vi "testclient.vi"() -> ()   [LabVIEW 2016]
uses:
  dllwrapper/tls data user event.ctl
  dllwrapper/tls new socket user event.ctl
  dllwrapper/async tls.lvlib
  lvasynctls.dll
panel:
  out "data 2":string
  out "data":string
  out "connection":u32
  out "errstring":string
  out "request type 3":u8 format="%.0x"
  out "request ID 3":u32 format="%.0x"
  out "error code 3":i32 format="%.0x"
  out "request type 2":u8 format="%.0x"
  out "request ID 2":u32 format="%.0x"
  out "error code 2":i32 format="%.0x"
  out "error code":i32
  out "request ID":u32 format="%.0x"
  out "request type":u32 format="%.0x"
  out "error out 10":errorcluster
  out "error out 9":errorcluster
  out "error out 6":errorcluster
  out "error out 5":errorcluster
  out "error out 4":errorcluster
  out "error out 3":errorcluster
  out "error out 2":errorcluster
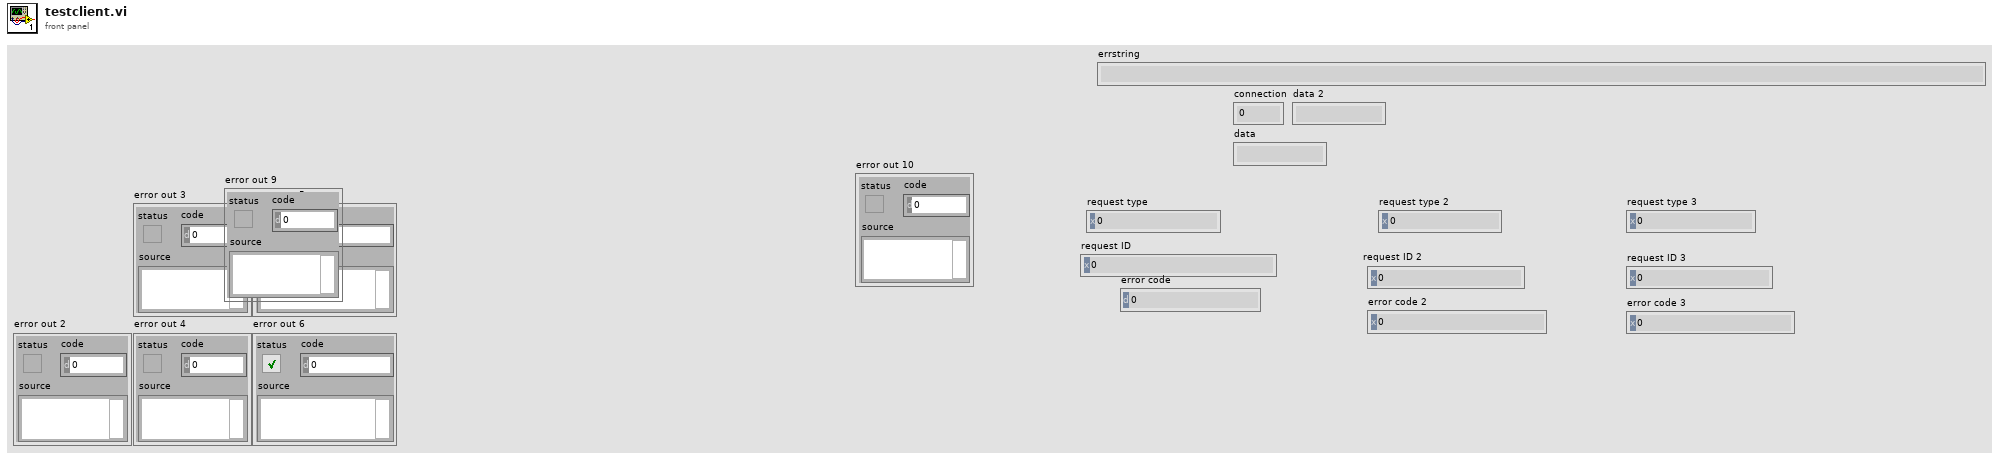
[diagram p1: front panel]
types:
  T1 = typedef "async tls.lvlib/tls new socket user event.ctl" = cluster{"request type":u32, "request ID":u32, "error code":i32, "errstring":string, "connection":u64}
  T2 = typedef "async tls.lvlib/tls data user event.ctl" = cluster{"request type":u8, "request ID":u32, "error code":i32, "data":string}
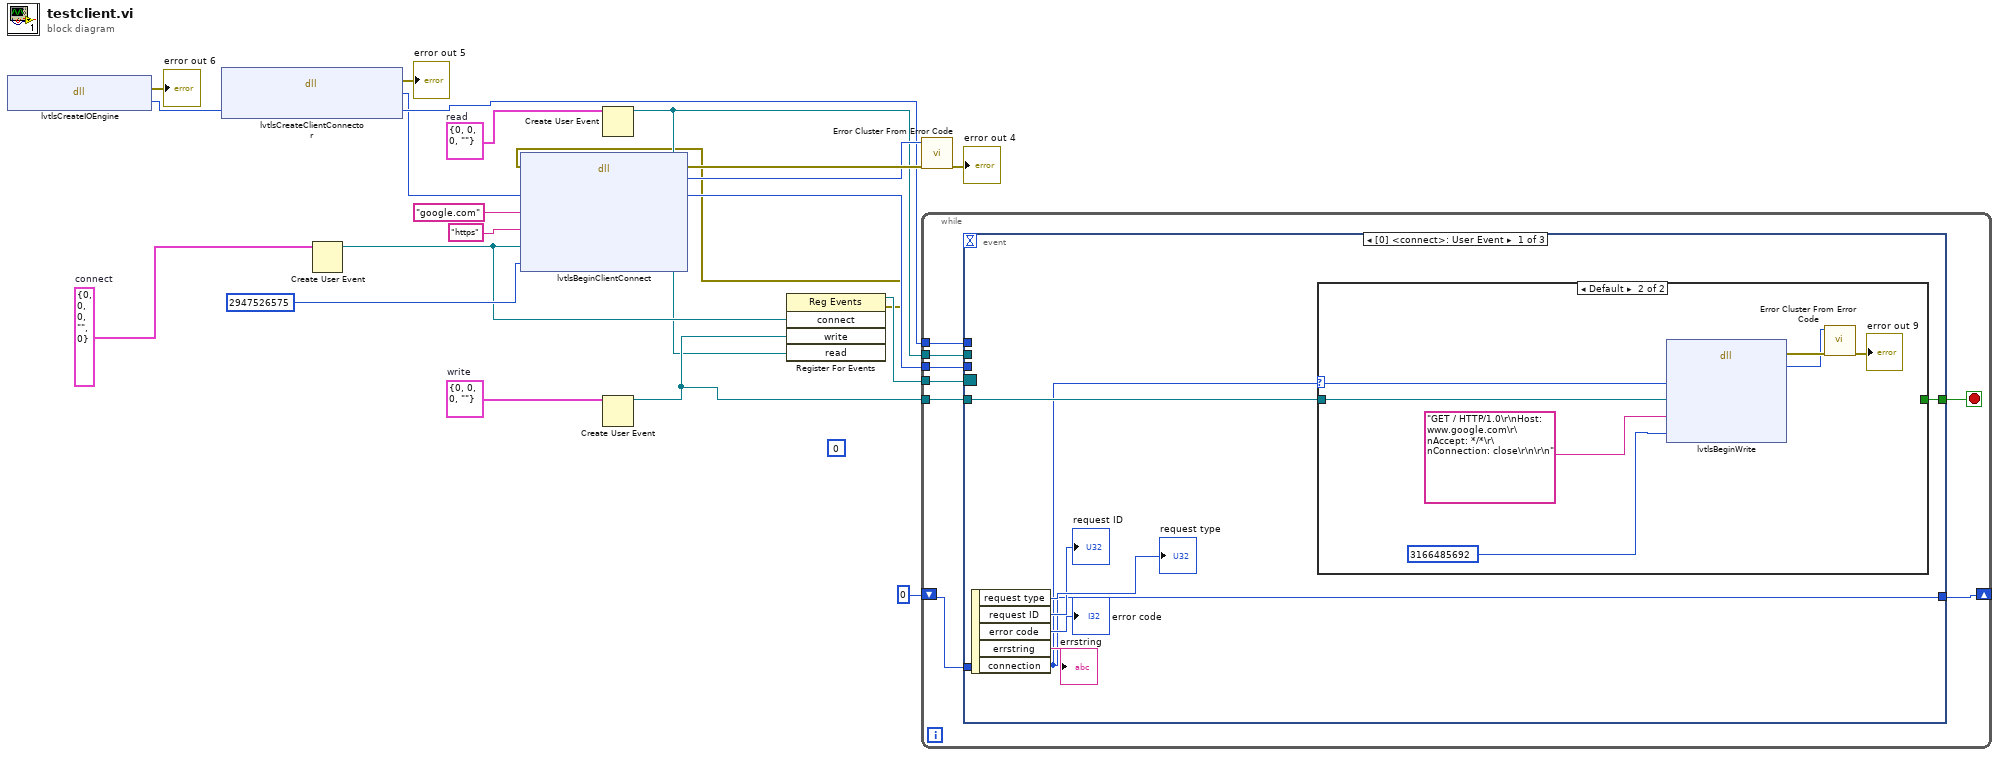
[diagram p0: block diagram]
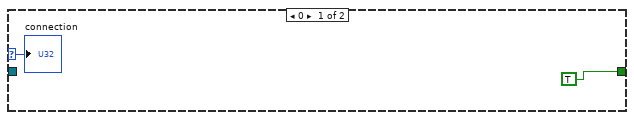
[diagram p2: hidden frame]
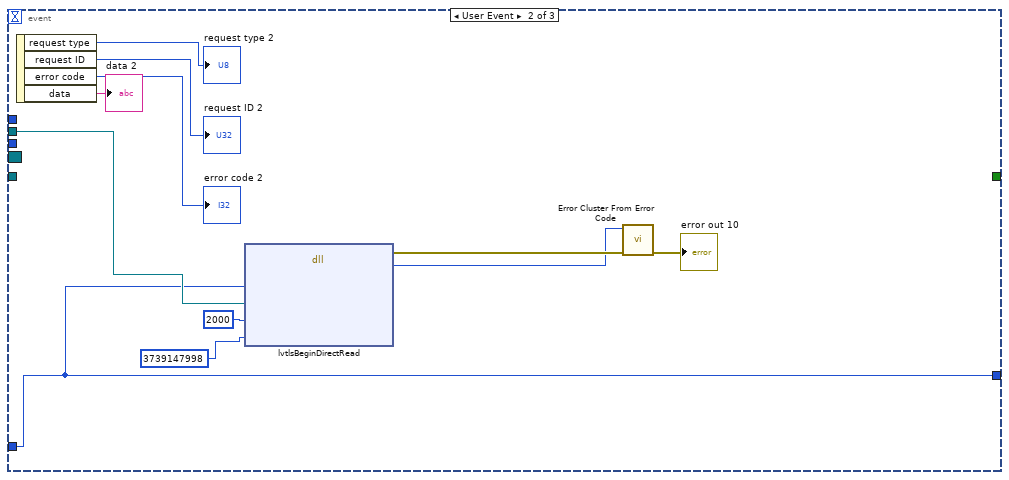
[diagram p3: hidden frame]
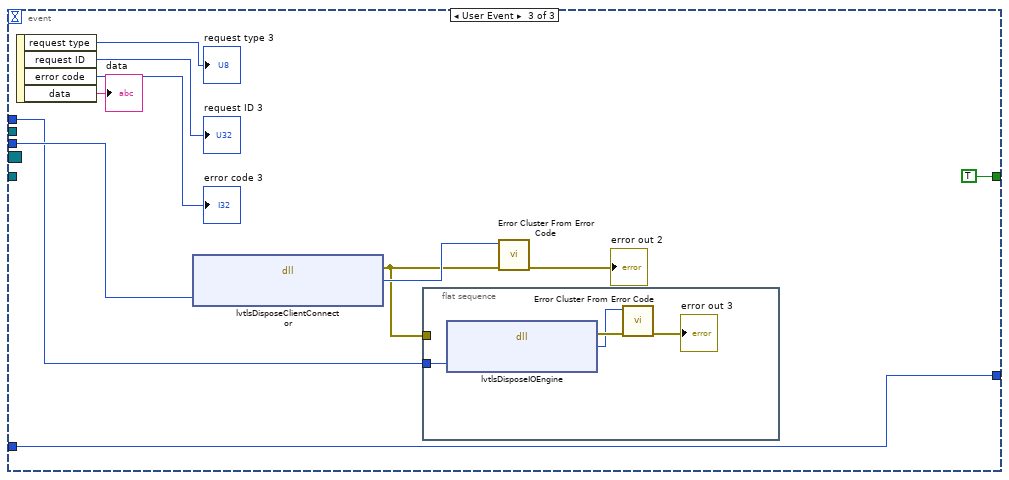
[diagram p4: hidden frame]
diagram:
  w3 = T1 {"request type"=0, "request ID"=0, "error code"=0, "errstring"="", "connection"=0}  # connect
  (unwired) u32 0 ("err")
  w13 = T2 {"request type"=0, "request ID"=0, "error code"=0, "data"=""}  # read
  w12 = T2 {"request type"=0, "request ID"=0, "error code"=0, "data"=""}  # write
  n1 = dll-call lib="C:/Users/IEUser/Desktop/libasynclvtls/lvasynctls.dll" fn="lvtlsCreateIOEngine"() -> (error out=→"error out 6":errorcluster, "engine"=w21:u64)  [unwired: 3 in, 1 out]
  n2 = dll-call lib="C:/Users/IEUser/Desktop/libasynclvtls/lvasynctls.dll" fn="lvtlsCreateClientConnector"("engine"=w21) -> (error out=→"error out 5":errorcluster, "client"=w8:u64, "engine"=w9:u64)  [unwired: 3 in, 1 out]
  n3 = Create User Event(user event datatype=w3) -> (user event=w6:refnum<user-event>)  [unwired: 1 in, 1 out]
  n4 = Create User Event(user event datatype=w13) -> (user event=w4:refnum<user-event>)  [unwired: 1 in, 1 out]
  n5 = Create User Event(user event datatype=w12) -> (user event=w5:refnum<user-event>)  [unwired: 1 in, 1 out]
  n6 = register-events(w6, w5, w4) -> (reference out=w14:refnum<event-registration>, error out=w1:errorcluster)  [unwired: 2 in]
  n7 = dll-call lib="C:/Users/IEUser/Desktop/libasynclvtls/lvasynctls.dll" fn="lvtlsBeginClientConnect"(error in=w1, "client"=w8, "host"="google.com", "port"="https", "event"=w6, "id"=u32 2947526575 ("err")) -> (error out=w17:errorcluster, "err"=w10:i32, "client"=w7:u64)  [unwired: 6 in, 1 out]
  n8 = call <vilib>:"Error Cluster From Error Code.vi"("error in (no error)"=w17, "error code (0)"=w10) -> ("error out"=→"error out 4":errorcluster)  [unwired: 7 in]
  n9 = while {
    tunnel: w14 -> [w29]
    tunnel: w5 -> [w27]
    tunnel: w7 -> [w26]
    tunnel: w4 -> [w25]
    tunnel: w9 -> [w24]
    shift-right: [w23] -> _
    shift-left: u32 0 -> [w22]
    stop <- w28 stop-if-true
    n10 = event shown="[0] <connect>: User Event" {
      selector: w29 -> [_ _ _]
      dyn-events: _ -> [_ _ _]
      timeout: _ -> [_ _ _]
      tunnel: [w30 _ TRUE] -> w28
      tunnel: w27 -> [w36 _ _]
      tunnel: w26 -> [_ _ w61]
      tunnel: w25 -> [_ w50 _]
      tunnel: w24 -> [_ _ w60]
      tunnel: [w31 w47 w58] -> w23
      tunnel: w22 -> [_ w47 w58]
      event User Event {
        n11 = event-data() -> ("request type"=→"request type":u32, "request ID"=→"request ID":u32, "error code"=→"error code":i32, "errstring"=→"errstring":string, "connection"=w31:u64)  [unwired: 1 in]
        n12 = case shown="Default" w31 {
          selector: w31 -> [w38 w39]
          tunnel: w36 -> [_ w41]
          tunnel: [TRUE _] -> w30
          frame 0 {
            "connection" <- w38
          }
          frame Default {
            n13 = dll-call lib="C:/Users/IEUser/Desktop/libasynclvtls/lvasynctls.dll" fn="lvtlsBeginWrite"("socket"=w39, "event"=w41, "data"="GET / HTTP/1.0\r\nHost: www.google.com\r\nAccept: */*\r\nConnection: close\r\n\r\n", "requestID"=u32 3166485692 ("err")) -> (error out=w45:errorcluster, "err"=w42:i32)  [unwired: 7 in, 1 out]
            n14 = call <vilib>:"Error Cluster From Error Code.vi"("error in (no error)"=w45, "error code (0)"=w42) -> ("error out"=→"error out 9":errorcluster)  [unwired: 7 in]
          }
        }
      }
      event User Event {
        n15 = event-data() -> ("request type"=→"request type 2":u8, "request ID"=→"request ID 2":u32, "error code"=→"error code 2":i32, "data"=→"data 2":string)  [unwired: 1 in]
        n16 = dll-call lib="C:/Users/IEUser/Desktop/libasynclvtls/lvasynctls.dll" fn="lvtlsBeginDirectRead"("socket"=w47, "event"=w50, "bytes to read"=2000, "id"=u32 3739147998 ("err")) -> (error out=w52:errorcluster, "err"=w49:i32)  [unwired: 7 in, 1 out]
        n17 = call <vilib>:"Error Cluster From Error Code.vi"("error in (no error)"=w52, "error code (0)"=w49) -> ("error out"=→"error out 10":errorcluster)  [unwired: 7 in]
      }
      event User Event {
        n18 = event-data() -> ("request type"=→"request type 3":u8, "request ID"=→"request ID 3":u32, "error code"=→"error code 3":i32, "data"=→"data":string)  [unwired: 1 in]
        n19 = dll-call lib="C:/Users/IEUser/Desktop/libasynclvtls/lvasynctls.dll" fn="lvtlsDisposeClientConnector"("client"=w61) -> (error out=w59:errorcluster, "err"=w63:i32)  [unwired: 4 in, 1 out]
        n20 = flat-sequence {
          tunnel: w60 -> [w68]
          tunnel: w59 -> [_]
          frame #0 {
            n21 = dll-call lib="C:/Users/IEUser/Desktop/libasynclvtls/lvasynctls.dll" fn="lvtlsDisposeIOEngine"("engine"=w68) -> (error out=w71:errorcluster, "err"=w70:i32)  [unwired: 4 in, 1 out]
            n22 = call <vilib>:"Error Cluster From Error Code.vi"("error in (no error)"=w71, "error code (0)"=w70) -> ("error out"=→"error out 3":errorcluster)  [unwired: 7 in]
          }
        }
        n23 = call <vilib>:"Error Cluster From Error Code.vi"("error in (no error)"=w59, "error code (0)"=w63) -> ("error out"=→"error out 2":errorcluster)  [unwired: 7 in]
      }
    }
  }
